vi "Header Exists.vi"(8 "error in":errorcluster, 10 "header":T1, 11 "session in":refnum<class "Session.lvclass">) -> (0 "error out":errorcluster, 1 "value":string, 2 "header exists?":bool, 3 "session out":refnum<class "Session.lvclass">)   [LabVIEW 2024, in "lib_NI_Advanced HTTP Client.lvlib" / "Session.lvclass"]
doc: "Determines if the header is associated with the HTTP session. Headers define attributes of the data exchanged between the client and server."
uses:
  Session.lvclass
  Header--Combo Box.ctl
  Session.lvclass/Session.ctl
  lvwebclient_64.dll
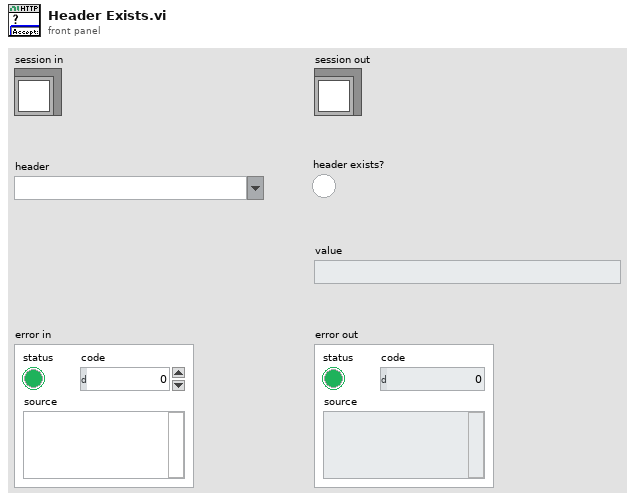
[diagram p1: front panel]
types:
  T1 = typedef "lib_NI_Advanced HTTP Client.lvlib/Session.lvclass/Header--Combo Box.ctl" = string
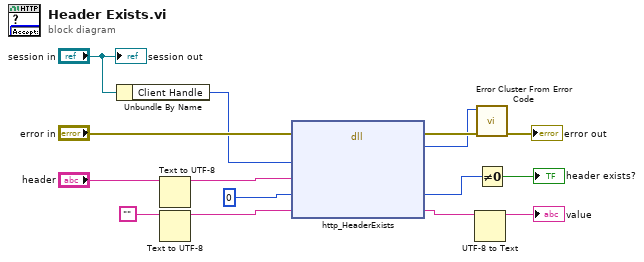
[diagram p0: block diagram]
diagram:
  n1 = Unbundle By Name("session in") -> ("Client Handle"=w7:u32)
  n2 = Text to UTF-8(11:"header") -> (3:w6:string)  [unwired: 2 in, 1 out]
  n3 = Text to UTF-8(11:"") -> (3:w5:string)  [unwired: 2 in, 1 out]
  n4 = dll-call lib="C:/Program Files/National Instruments/LabVIEW 2024/vi.lib/NI/Advanced HTTP Client/lvwebclient_*.*" fn="http_HeaderExists"(error in="error in", "handle"=w7, "headerName"=w6, "headerExists"=u32 0, "headerValue"=w5) -> (error out=w9:errorcluster, "return"=w8:i32, "headerExists"=w1:u32, "headerValue"=w3:string)  [unwired: 4 in, 1 out]
  n5 = UTF-8 to Text(11:w3) -> (3:→"value":string)  [unwired: 2 in, 1 out]
  n6 = call "Error Cluster From Error Code.vi"("error in (no error)"=w9, "error code (0)"=w8) -> ("error out"=→"error out":errorcluster)  [unwired: 7 in]
  n7 = Not Equal To 0?(x=w1) -> (x != 0?=→"header exists?":bool)
  "session out" <- "session in"
